vi "Find Edge Parameter.vi"(7 "Action":T6, 8 "error in (no error)":errorcluster, 9 "Line Fit Options in":T4={"Number of Lines"=1, "Type"=enum."First Edge Rake", "Min. Score"=10.0, "Max. Score"=1000.0, "Orientation"=0.0, "Angle Range"=45.0, "Angle Tolerance"=1.0, "Step Size"=7, "Min. SNR (db)"=0.0, "Min. Points (%)"=25.0, "Hough Iterations"=5} {"Min. Points (%)" min=0.0 max=100.0; "Min. SNR (db)" min=0.0; "Max. Score" min=0.0 max=1024.0; "Min. Score" min=0.0 max=1024.0 step=1.0}, 10 "Options in":T3={"Search Direction"=0, "Edge Options"={"Edge Polarity"=0, "Kernel Size"=3, "Width"=3, "Minimum Edge Strength"=10.0, "Interpolation Type"=enum."Bilinear Fixed", "Data Processing Method"=enum."Average"}, "Show Search Area"=FALSE, "Show Search Lines"=FALSE, "Show Edges Found"=FALSE, "Show Result"=TRUE, "Search Area Color"=65280, "Search Lines Color"=255, "Edge Locations Color"=16776960, "Result Color"=16711680, "Overlay Group Name"=""} {"Edge Options"."Edge Polarity" items=["All Edges", "Rising Edges", "Falling Edges"]; "Edge Options"."Minimum Edge Strength" format="%.2f"; "Edge Options"."Width" step=2; "Edge Options"."Kernel Size" step=2; "Search Direction" items=["Left to Right", "Right to Left", "Top to Bottom", "Bottom to Top"]}, 11 "Directory":string) -> (0 "error out":errorcluster, 2 "Line Fit Options out":T4={"Number of Lines"=1, "Type"=enum."First Edge Rake", "Min. Score"=10.0, "Max. Score"=1000.0, "Orientation"=0.0, "Angle Range"=45.0, "Angle Tolerance"=1.0, "Step Size"=7, "Min. SNR (db)"=0.0, "Min. Points (%)"=25.0, "Hough Iterations"=5} {"Min. Points (%)" min=0.0 max=100.0; "Min. SNR (db)" min=0.0; "Max. Score" min=0.0 max=1024.0; "Min. Score" min=0.0 max=1024.0 step=1.0}, 3 "Options out":T3={"Search Direction"=0, "Edge Options"={"Edge Polarity"=0, "Kernel Size"=3, "Width"=3, "Minimum Edge Strength"=10.0, "Interpolation Type"=enum."Bilinear Fixed", "Data Processing Method"=enum."Average"}, "Show Search Area"=FALSE, "Show Search Lines"=FALSE, "Show Edges Found"=FALSE, "Show Result"=TRUE, "Search Area Color"=65280, "Search Lines Color"=255, "Edge Locations Color"=16776960, "Result Color"=16711680, "Overlay Group Name"=""} {"Edge Options"."Edge Polarity" items=["All Edges", "Rising Edges", "Falling Edges"]; "Edge Options"."Minimum Edge Strength" format="%.2f"; "Edge Options"."Width" step=2; "Edge Options"."Kernel Size" step=2; "Search Direction" items=["Left to Right", "Right to Left", "Top to Bottom", "Bottom to Top"]})   [LabVIEW 2017, in "File.lvlib"]
uses:
  File.lvlib
  <vilib>/vision/Measure.llb/Edge Polarity.ctl
  <vilib>/vision/Measure.llb/Edge Options.ctl
  <vilib>/vision/Measure.llb/Straight Edge Process.ctl
  <vilib>/vision/Measure.llb/Straight Edge Options.ctl
  <vilib>/Utility/config.llb/NI_LVConfig.lvlib
  <vilib>/Utility/config.llb/Config Data RefNum.ctl
  <vilib>/Utility/config.llb/Read Key (Boolean).vi
  <vilib>/Utility/config.llb/Read Key (Double).vi
  <vilib>/Utility/config.llb/Read Key (U32).vi
  <vilib>/Utility/config.llb/Read Key (String).vi
  <vilib>/Utility/config.llb/Write Key (Boolean).vi
  <vilib>/Utility/config.llb/Write Key (Double).vi
  <vilib>/Utility/config.llb/Write Key (U32).vi
  <vilib>/Utility/config.llb/Write Key (String).vi
  Control/File Action.ctl
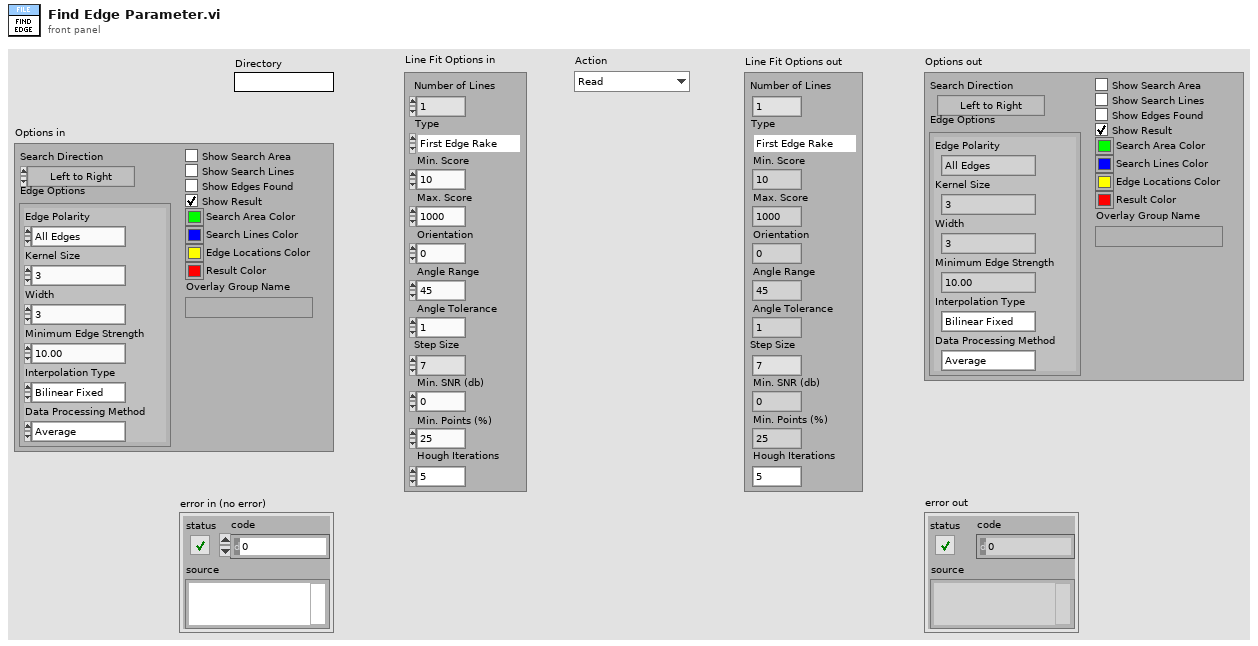
[diagram p1: front panel]
types:
  T1 = typedef "Edge Options.ctl" = cluster{"Edge Polarity":T2, "Kernel Size":u32, "Width":u32, "Minimum Edge Strength":sgl, "Interpolation Type":enum32{"Zero Order", "Bilinear", "Quadratic", "Cubic", "Bilinear Fixed"}, "Data Processing Method":enum32{"Average", "Median"}}
  T2 = typedef "Edge Polarity.ctl" = u32
  T3 = cluster{"Search Direction":u32, "Edge Options":T1, "Show Search Area":bool, "Show Search Lines":bool, "Show Edges Found":bool, "Show Result":bool, "Search Area Color":u32, "Search Lines Color":u32, "Edge Locations Color":u32, "Result Color":u32, "Overlay Group Name":string}
  T4 = typedef "Straight Edge Options.ctl" = cluster{"Number of Lines":i32, "Type":T5, "Min. Score":dbl, "Max. Score":dbl, "Orientation":dbl, "Angle Range":dbl, "Angle Tolerance":dbl, "Step Size":u32, "Min. SNR (db)":dbl, "Min. Points (%)":dbl, "Hough Iterations":i32}
  T5 = typedef "Straight Edge Process.ctl" = enum32{"First Edge Rake", "Best Edge Rake", "Hough Edge Rake", "First Edge Projection", "Best Edge Projection"}
  T6 = typedef "File.lvlib/File Action.ctl" = enum16{"Read", "Write"}
  T7 = typedef "NI_LVConfig.lvlib/Config Data RefNum.ctl" = refnum<k1>
  T8 = cluster{"Config refnum":T7, "Options":cluster{"Search Direction":u32, "Edge Options":T1, "Show Search Area":bool, "Show Search Lines":bool, "Show Edges Found":bool, "Show Result":bool, "Search Area Color":u32, "Search Lines Color":u32, "Edge Locations Color":u32, "Result Color":u32, "Overlay Group Name":string}, "Line Fit Options":T4, "Section":cluster{"Options":string, "Line Fit Options":string}}
  T9 = enum32{"Zero Order", "Bilinear", "Quadratic", "Cubic", "Bilinear Fixed"}
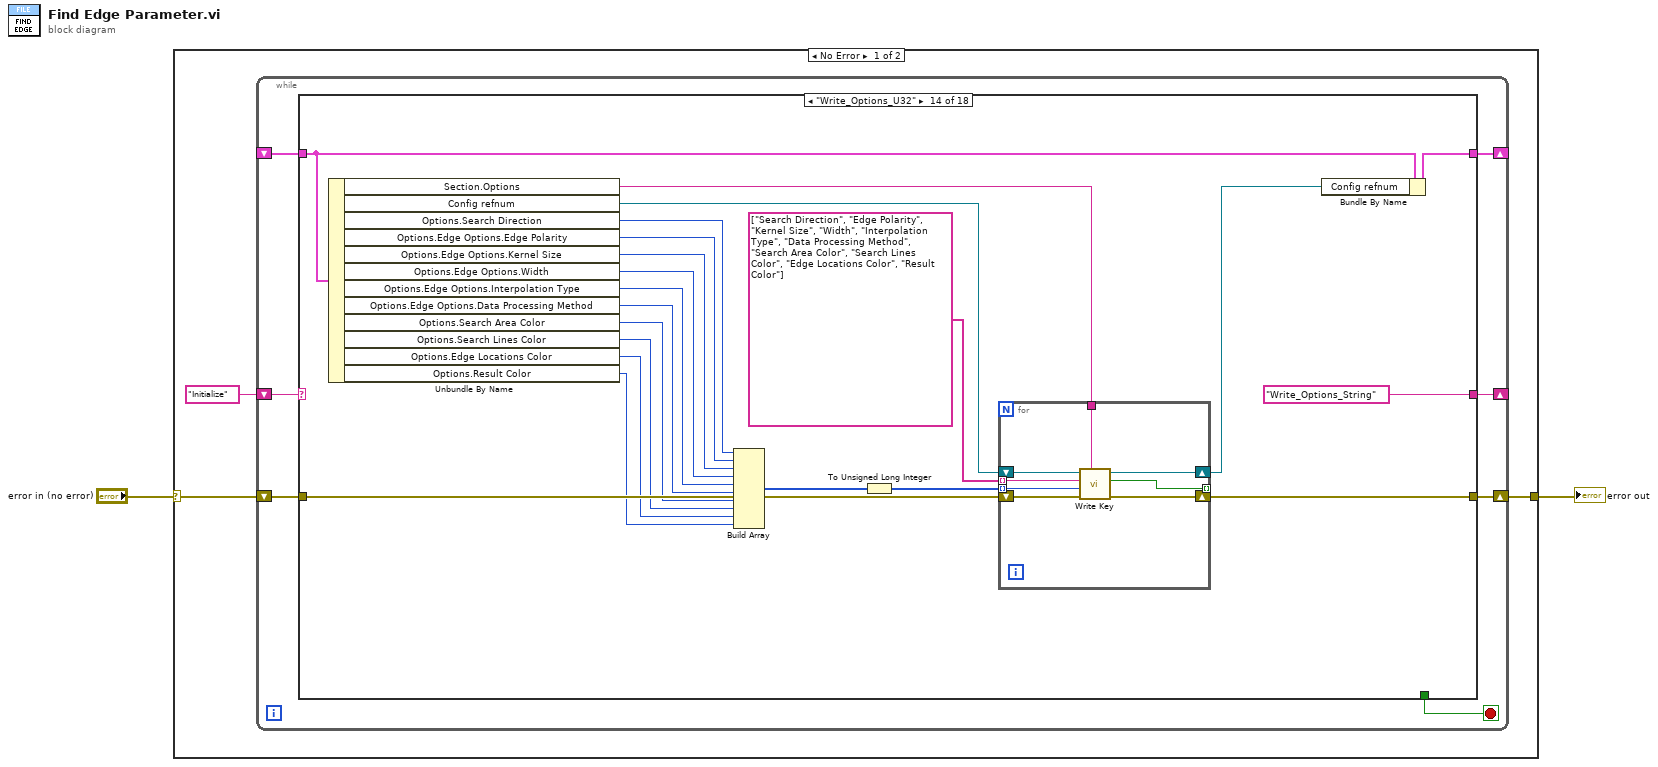
[diagram p0: block diagram]
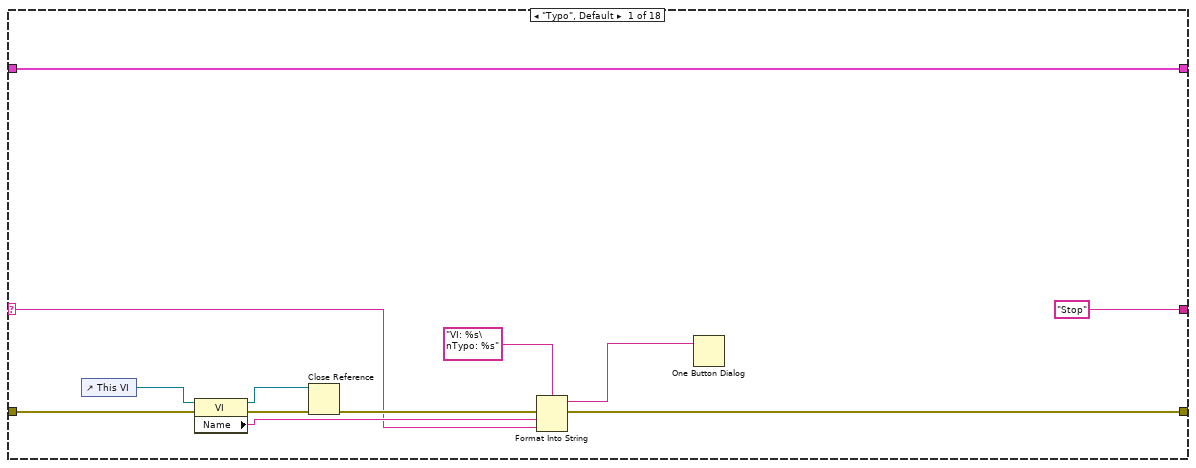
[diagram p2: hidden frame]
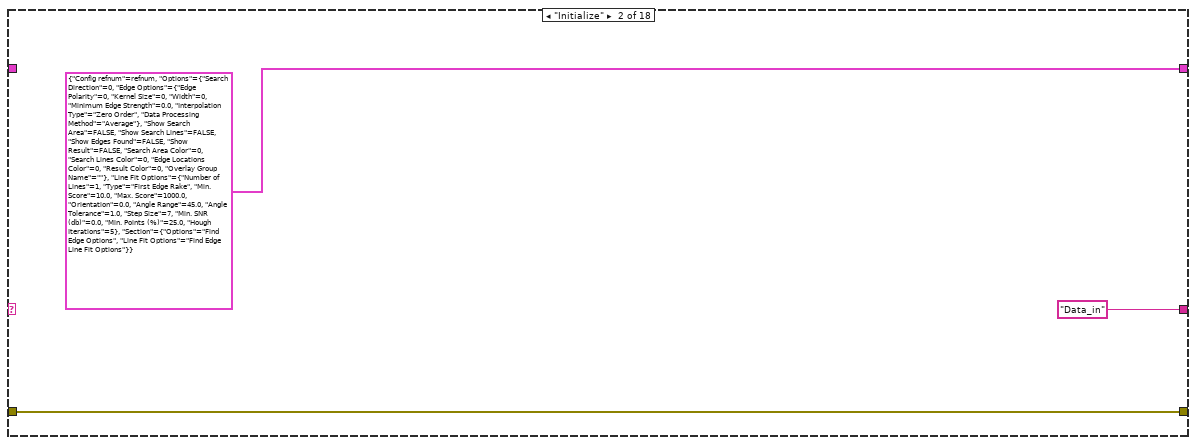
[diagram p3: hidden frame]
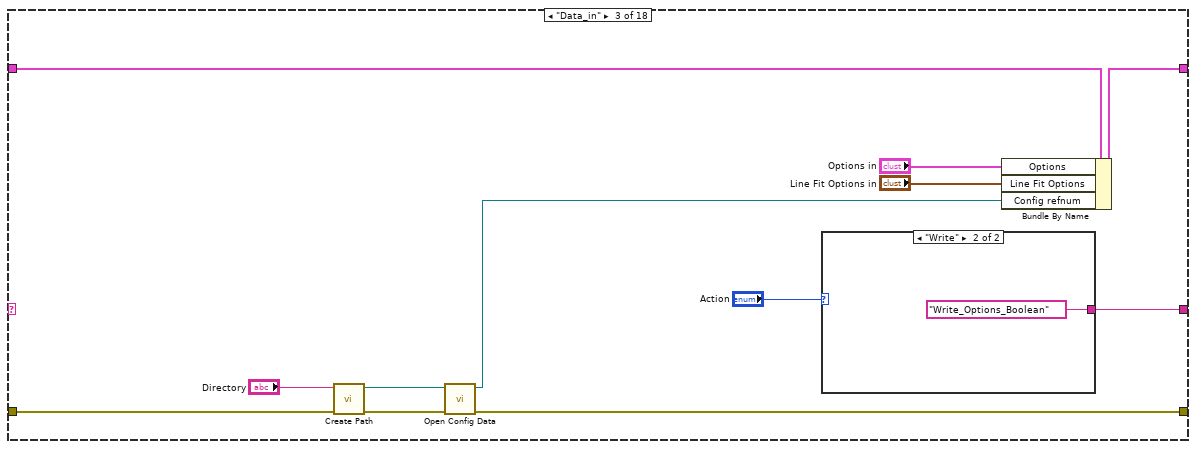
[diagram p4: hidden frame]
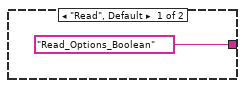
[diagram p5: hidden frame]
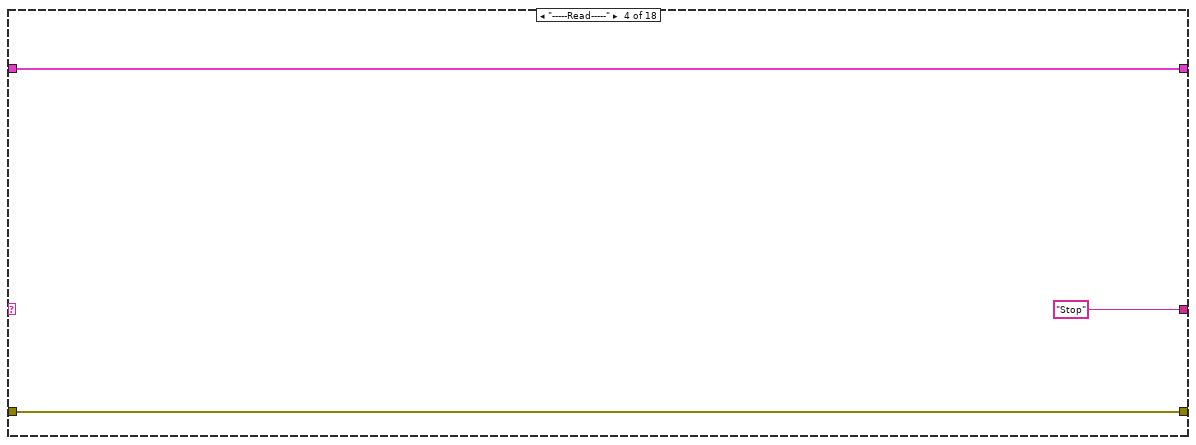
[diagram p6: hidden frame]
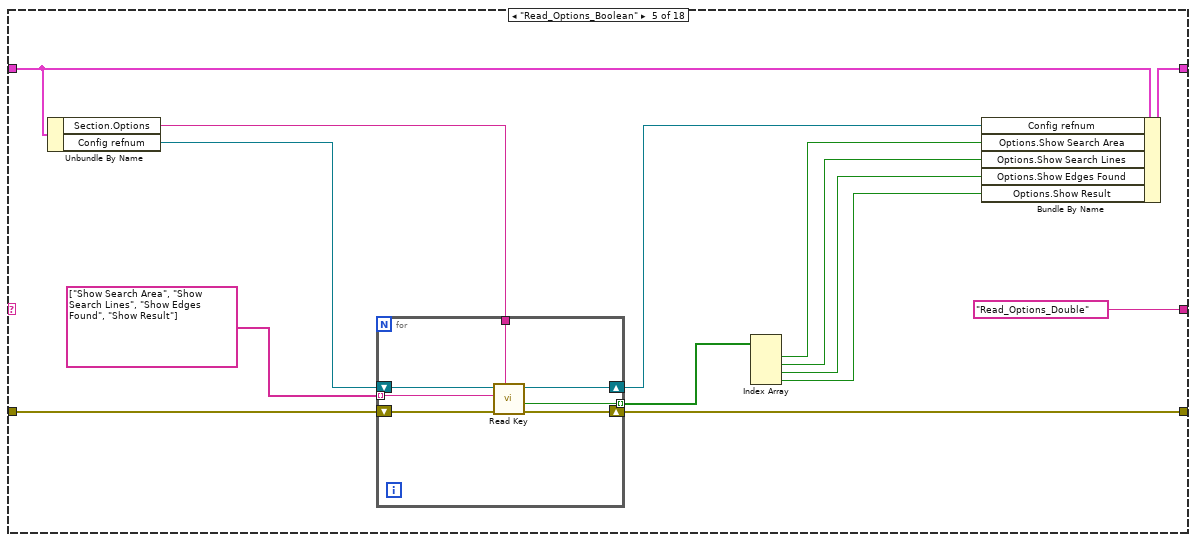
[diagram p7: hidden frame]
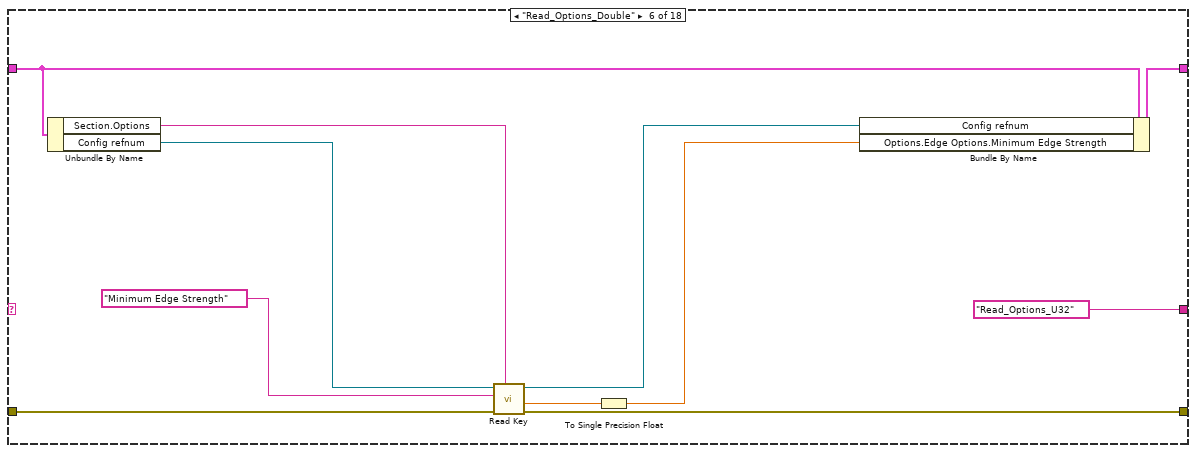
[diagram p8: hidden frame]
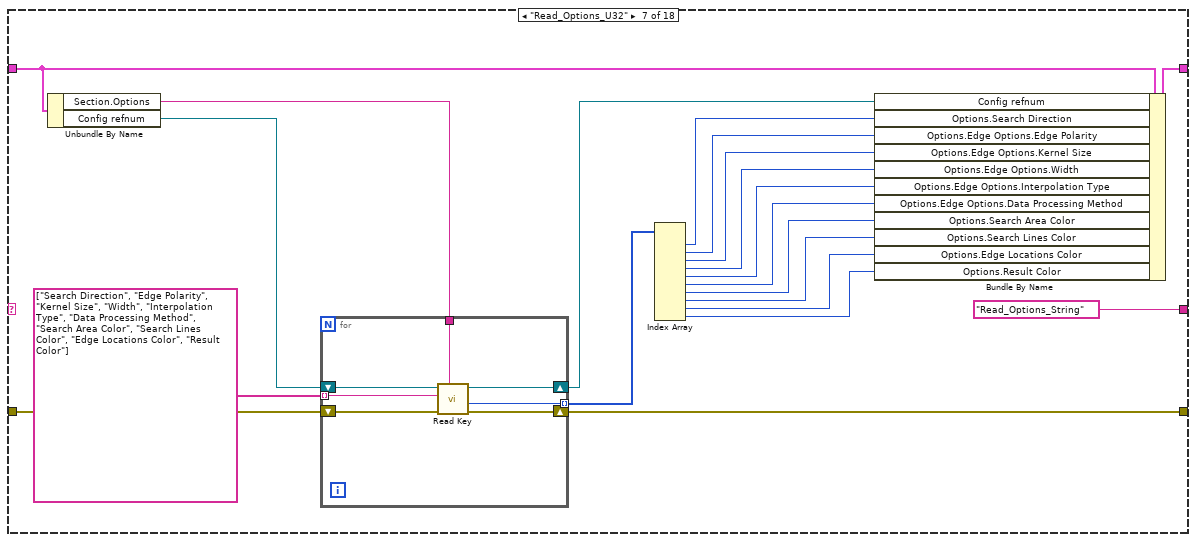
[diagram p9: hidden frame]
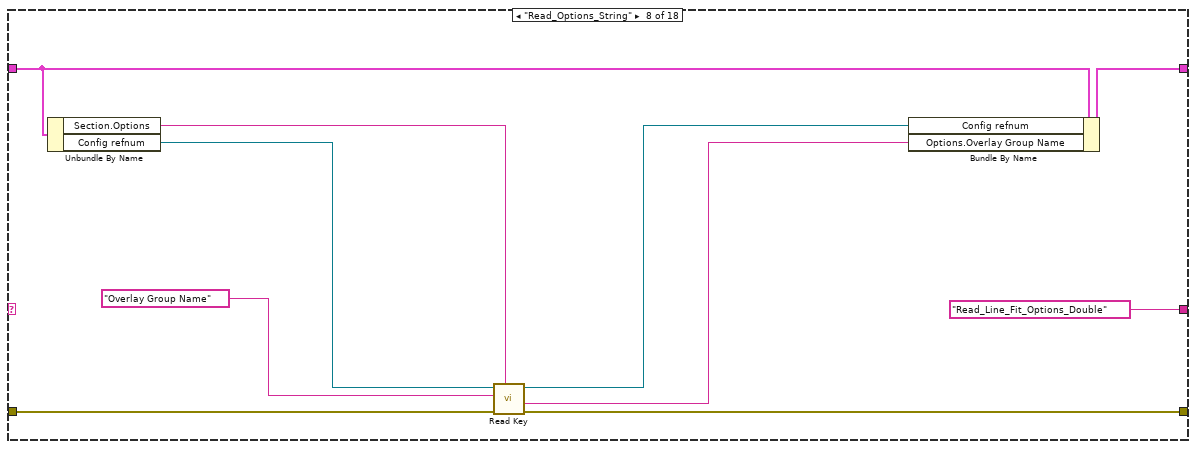
[diagram p10: hidden frame]
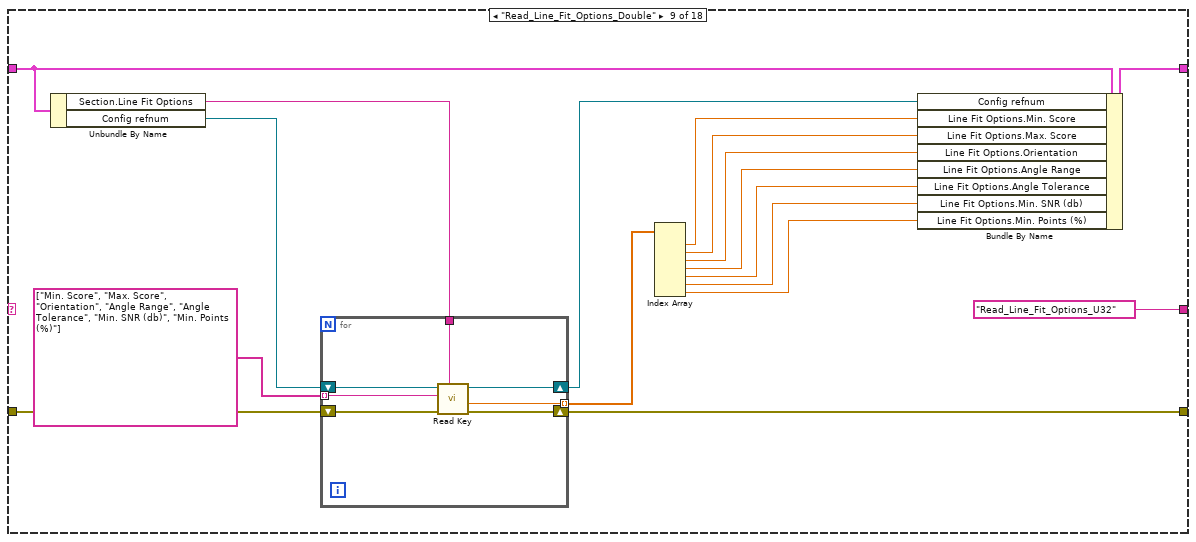
[diagram p11: hidden frame]
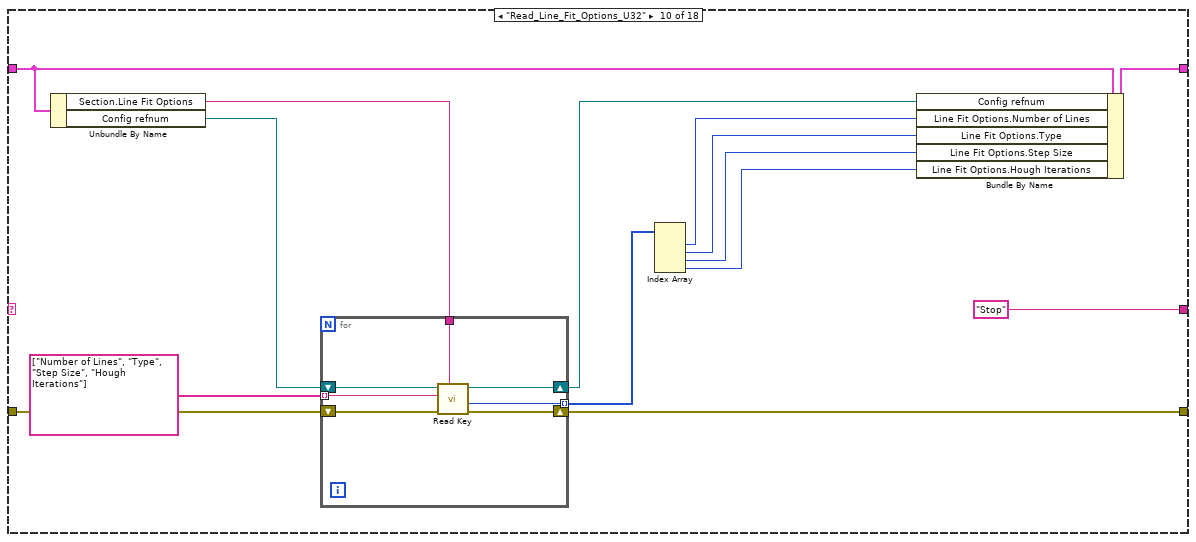
[diagram p12: hidden frame]
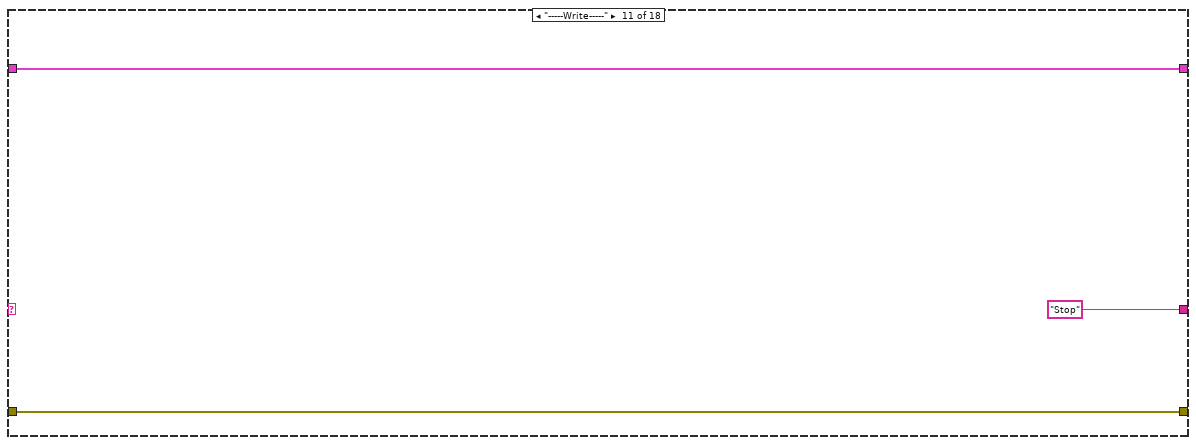
[diagram p13: hidden frame]
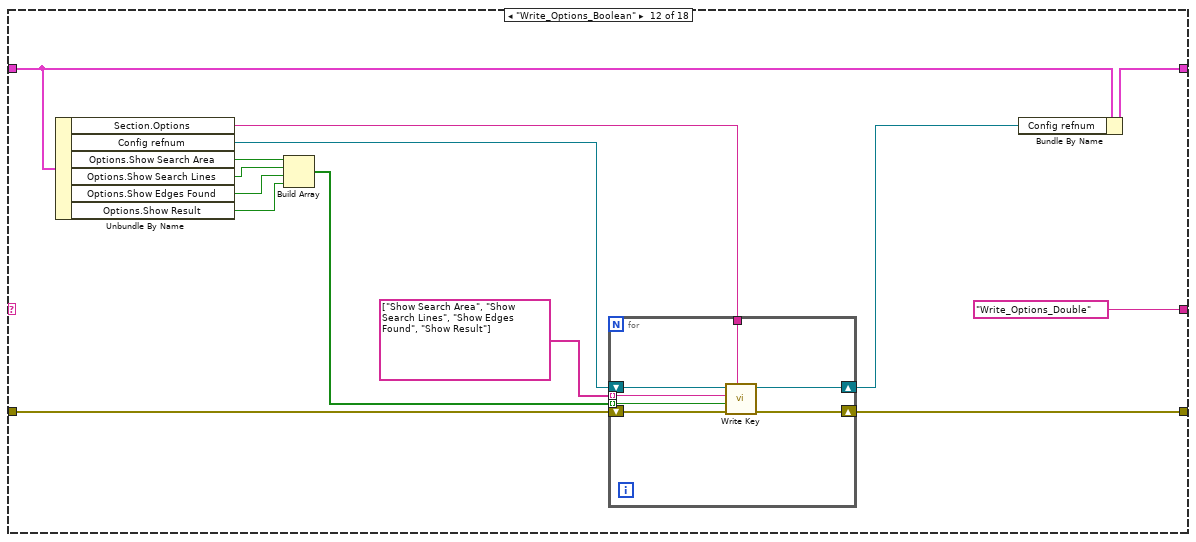
[diagram p14: hidden frame]
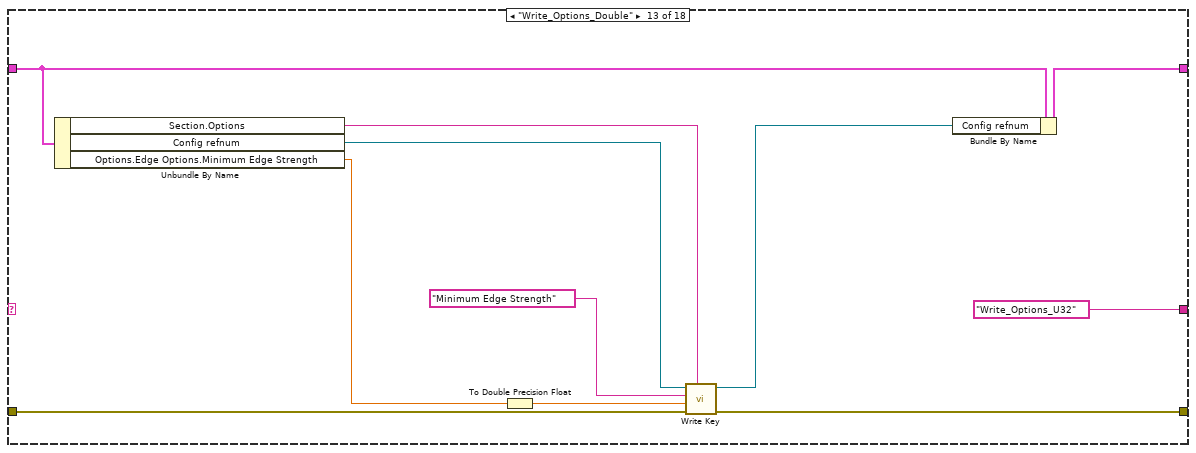
[diagram p15: hidden frame]
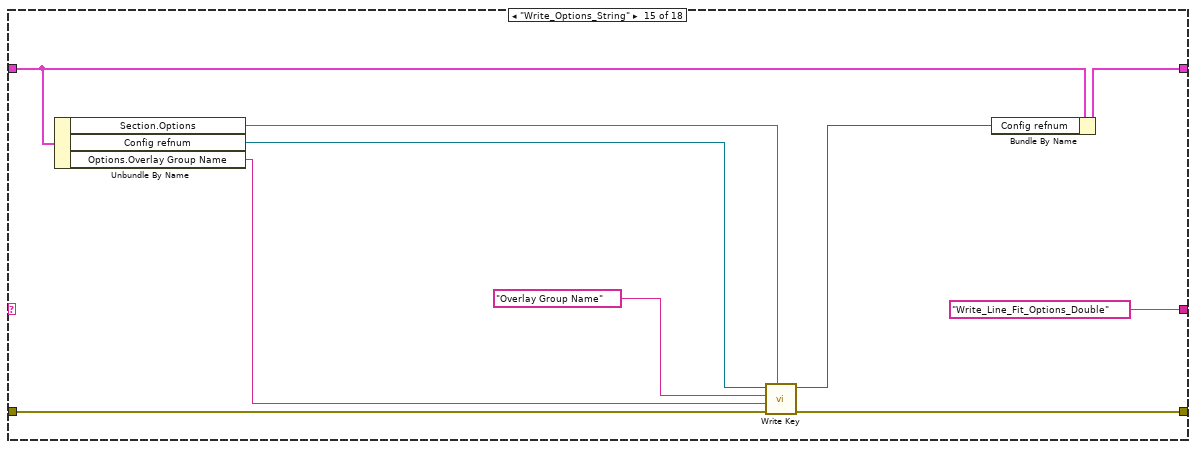
[diagram p16: hidden frame]
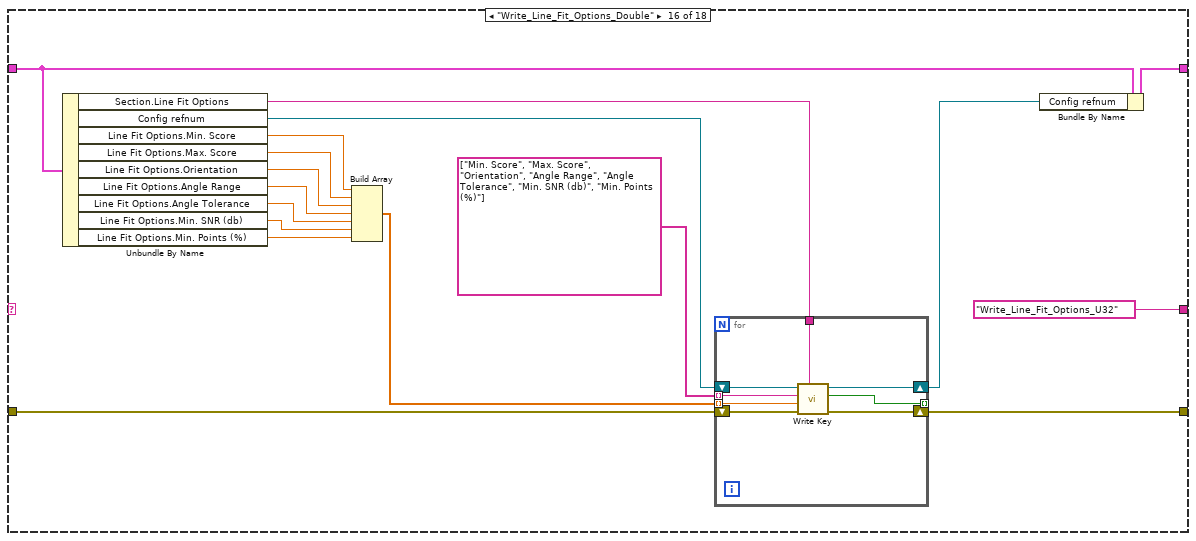
[diagram p17: hidden frame]
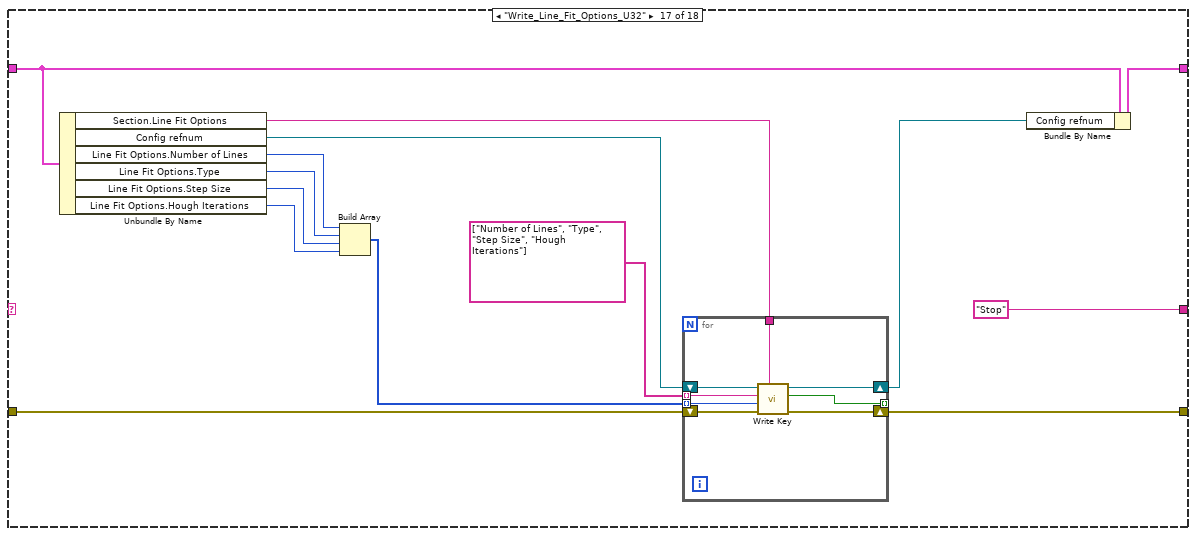
[diagram p18: hidden frame]
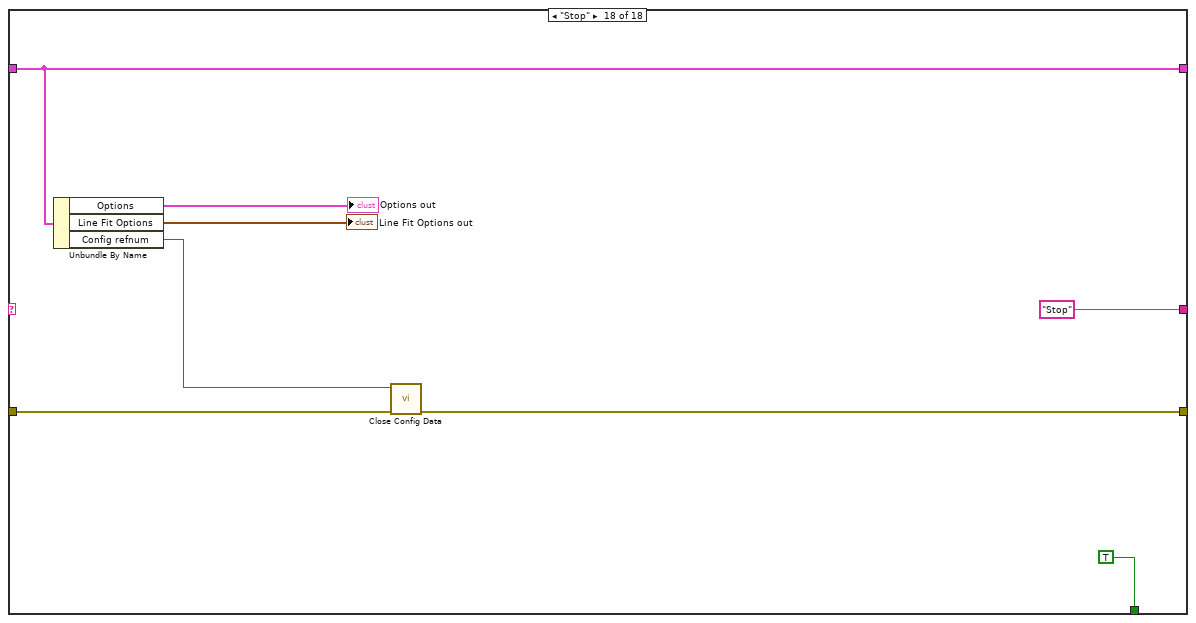
[diagram p19: hidden frame]
diagram:
  n1 = case shown="No Error" "error in (no error)" {
    selector: "error in (no error)" -> [w5 w288]
    tunnel: [w3 w288] -> w1
    frame No Error {
      n2 = while {
        shift-right: [w10] -> w3
        shift-left: w5 -> [w11]
        shift-right: [w9] -> _
        shift-left: "Initialize" -> [w12]
        shift-right: [w7] -> _
        shift-left: _ -> [w6]
        stop <- w8 stop-if-true
        n3 = case shown="\"Write_Options_U32\"" w12 {
          selector: w12 -> [w16 _ _ _ _ _ _ _ _ _ _ _ _ _ _ _ _ _]
          tunnel: w11 -> [w24 w26 w39 w44 w58 w76 w96 w113 w130 w151 w161 w175 w193 w214 w232 w249 w271 w285]
          tunnel: [w21 w26 w34 w44 w56 w74 w94 w111 w128 w149 w161 w173 w191 w212 w230 w247 w269 w283] -> w10
          tunnel: ["Stop" "Data_in" w36 "Stop" "Read_Options_Double" "Read_Options_U32" "Read_Options_String" "Read_Line_Fit_Options_Double" "Read_Line_Fit_Options_U32" "Stop" "Stop" "Write_Options_Double" "Write_Options_U32" "Write_Options_String" "Write_Line_Fit_Options_Double" "Write_Line_Fit_Options_U32" "Stop" "Stop"] -> w9
          tunnel: [_ _ _ _ _ _ _ _ _ _ _ _ _ _ _ _ _ TRUE] -> w8
          tunnel: [w13 T8 {"Config refnum"=refnum, "Options"={"Search Direction"=0, "Edge Options"={"Edge Polarity"=0, "Kernel Size"=0, "Width"=0, "Minimum Edge Strength"=0.0, "Interpolation Type"=enum."Zero Order", "Data Processing Method"=enum."Average"}, "Show Search Area"=FALSE, "Show Search Lines"=FALSE, "Show Edges Found"=FALSE, "Show Result"=FALSE, "Search Area Color"=0, "Search Lines Color"=0, "Edge Locations Color"=0, "Result Color"=0, "Overlay Group Name"=""}, "Line Fit Options"={"Number of Lines"=1, "Type"=enum."First Edge Rake", "Min. Score"=10.0, "Max. Score"=1000.0, "Orientation"=0.0, "Angle Range"=45.0, "Angle Tolerance"=1.0, "Step Size"=7, "Min. SNR (db)"=0.0, "Min. Points (%)"=25.0, "Hough Iterations"=5}, "Section"={"Options"="Find Edge Options", "Line Fit Options"="Find Edge Line Fit Options"}} w37 w43 w51 w70 w89 w107 w123 w144 w160 w169 w187 w208 w226 w243 w265 w284] -> w7
          tunnel: w6 -> [w13 _ w38 w43 w57 w75 w95 w112 w129 w150 w160 w174 w192 w213 w231 w248 w270 w284]
          frame "Typo", Default {
            n4 = control-ref of="This VI"() -> (w22:refnum<vi>)
            n5 = property class="VI"(reference=w22, error in=w24) -> (reference out=w17:refnum<vi>, error out=w23:errorcluster, "Name"=w19:string)
            n6 = Close Reference(reference=w17, error in (no error)=w23) -> (error out=w18:errorcluster)
            n7 = Format Into String(format string="VI: %s\nTypo: %s", error in=w18, w19, w16) -> (resulting string=w15:string, error out=w21:errorcluster)  [unwired: 1 in]
            n8 = One Button Dialog(message=w15) -> ()  [unwired: 1 in, 1 out]
          }
          frame "Initialize" {
          }
          frame "Data_in" {
            n9 = call "Create Path.vi"("error in (no error)"=w39, "Directory"="Directory") -> ("error out"=w35:errorcluster, "Path"=w33:path)  [unwired: 8 in]
            n10 = call <vilib>:"Open Config Data.vi"("error in (no error)"=w35, "configuration file path"=w33) -> ("error out"=w34:errorcluster, "refnum"=w31:T7)  [unwired: 7 in, 1 out]
            n11 = case shown="\"Write\"" "Action" {
              tunnel: ["Read_Options_Boolean" "Write_Options_Boolean"] -> w36
              frame "Read", Default {
              }
              frame "Write" {
              }
            }
            n12 = Bundle By Name(cluster=w38, "Options"="Options in", "Line Fit Options"="Line Fit Options in", "Config refnum"=w31) -> (w37:T8)
          }
          frame "-----Read-----" {
          }
          frame "Read_Options_Boolean" {
            n13 = Unbundle By Name(w57) -> ("Section.Options"=w55:string, "Config refnum"=w54:T7)
            n14 = for {
              tunnel: w55 -> [w63]
              shift-right: [w64] -> w56
              shift-left: w58 -> [w65]
              shift-right: [w61] -> w50
              shift-left: w54 -> [w62]
              tunnel: string[] ["Show Search Area", "Show Search Lines", "Show Edges Found", "Show Result"] -> [w60] mode=indexing
              tunnel: [w59] -> w52 mode=indexing
              n15 = call-poly <vilib>:"Read Key.vi"("section"=w63, "error in (no error)"=w65, "key"=w60, "refnum"=w62) -> ("error out"=w64:errorcluster, "value"=w59:bool, "refnum out"=w61:T7)  [unwired: 4 in, 1 out]
            }
            n16 = Index Array(array=w52) -> (element #1=w49:bool, element #2=w48:bool, element #3=w47:bool, element #4=w46:bool)  [unwired: 4 in]
            n17 = Bundle By Name(cluster=w57, "Config refnum"=w50, "Options.Show Search Area"=w49, "Options.Show Search Lines"=w48, "Options.Show Edges Found"=w47, "Options.Show Result"=w46) -> (w51:T8)
          }
          frame "Read_Options_Double" {
            n18 = Unbundle By Name(w75) -> ("Section.Options"=w73:string, "Config refnum"=w72:T7)
            n19 = call-poly <vilib>:"Read Key.vi"("section"=w73, "error in (no error)"=w76, "key"="Minimum Edge Strength", "refnum"=w72) -> ("error out"=w74:errorcluster, "value"=w67:dbl, "refnum out"=w69:T7)  [unwired: 4 in, 1 out]
            n20 = To Single Precision Float(number=w67) -> (single precision float=w66:sgl)
            n21 = Bundle By Name(cluster=w75, "Config refnum"=w69, "Options.Edge Options.Minimum Edge Strength"=w66) -> (w70:T8)
          }
          frame "Read_Options_U32" {
            n22 = Unbundle By Name(w95) -> ("Section.Options"=w93:string, "Config refnum"=w92:T7)
            n23 = for {
              tunnel: w93 -> [w101]
              shift-right: [w102] -> w94
              shift-left: w96 -> [w103]
              shift-right: [w99] -> w88
              shift-left: w92 -> [w100]
              tunnel: string[] ["Search Direction", "Edge Polarity", "Kernel Size", "Width", "Interpolation Type", "Data Processing Method", "Search Area Color", "Search Lines Color", "Edge Locations Color", "Result Color"] -> [w98] mode=indexing
              tunnel: [w97] -> w90 mode=indexing
              n24 = call-poly <vilib>:"Read Key.vi"("section"=w101, "error in (no error)"=w103, "key"=w98, "refnum"=w100) -> ("error out"=w102:errorcluster, "value"=w97:u32, "refnum out"=w99:T7)  [unwired: 4 in, 1 out]
            }
            n25 = Index Array(array=w90) -> (element #1=w87:u32, element #2=w86:u32, element #3=w85:u32, element #4=w84:u32, element #5=w82:u32, element #6=w81:u32, element #7=w80:u32, element #8=w79:u32, element #9=w78:u32, element #10=w77:u32)  [unwired: 10 in]
            n26 = Bundle By Name(cluster=w95, "Config refnum"=w88, "Options.Search Direction"=w87, "Options.Edge Options.Edge Polarity"=w86, "Options.Edge Options.Kernel Size"=w85, "Options.Edge Options.Width"=w84, "Options.Edge Options.Interpolation Type"=w82, "Options.Edge Options.Data Processing Method"=w81, "Options.Search Area Color"=w80, "Options.Search Lines Color"=w79, "Options.Edge Locations Color"=w78, "Options.Result Color"=w77) -> (w89:T8)
          }
          frame "Read_Options_String" {
            n27 = Unbundle By Name(w112) -> ("Section.Options"=w110:string, "Config refnum"=w109:T7)
            n28 = call-poly <vilib>:"Read Key.vi"("section"=w110, "error in (no error)"=w113, "key"="Overlay Group Name", "refnum"=w109) -> ("error out"=w111:errorcluster, "value"=w104:string, "refnum out"=w106:T7)  [unwired: 4 in, 1 out]
            n29 = Bundle By Name(cluster=w112, "Config refnum"=w106, "Options.Overlay Group Name"=w104) -> (w107:T8)
          }
          frame "Read_Line_Fit_Options_Double" {
            n30 = Unbundle By Name(w129) -> ("Section.Line Fit Options"=w127:string, "Config refnum"=w126:T7)
            n31 = for {
              tunnel: w127 -> [w135]
              shift-right: [w136] -> w128
              shift-left: w130 -> [w137]
              shift-right: [w133] -> w122
              shift-left: w126 -> [w134]
              tunnel: string[] ["Min. Score", "Max. Score", "Orientation", "Angle Range", "Angle Tolerance", "Min. SNR (db)", "Min. Points (%)"] -> [w132] mode=indexing
              tunnel: [w131] -> w124 mode=indexing
              n32 = call-poly <vilib>:"Read Key.vi"("section"=w135, "error in (no error)"=w137, "key"=w132, "refnum"=w134) -> ("error out"=w136:errorcluster, "value"=w131:dbl, "refnum out"=w133:T7)  [unwired: 4 in, 1 out]
            }
            n33 = Index Array(array=w124) -> (element #1=w121:dbl, element #2=w120:dbl, element #3=w119:dbl, element #4=w118:dbl, element #5=w116:dbl, element #6=w115:dbl, element #7=w114:dbl)  [unwired: 7 in]
            n34 = Bundle By Name(cluster=w129, "Config refnum"=w122, "Line Fit Options.Min. Score"=w121, "Line Fit Options.Max. Score"=w120, "Line Fit Options.Orientation"=w119, "Line Fit Options.Angle Range"=w118, "Line Fit Options.Angle Tolerance"=w116, "Line Fit Options.Min. SNR (db)"=w115, "Line Fit Options.Min. Points (%)"=w114) -> (w123:T8)
          }
          frame "Read_Line_Fit_Options_U32" {
            n35 = Unbundle By Name(w150) -> ("Section.Line Fit Options"=w148:string, "Config refnum"=w147:T7)
            n36 = for {
              tunnel: w148 -> [w156]
              shift-right: [w157] -> w149
              shift-left: w151 -> [w158]
              shift-right: [w154] -> w143
              shift-left: w147 -> [w155]
              tunnel: string[] ["Number of Lines", "Type", "Step Size", "Hough Iterations"] -> [w153] mode=indexing
              tunnel: [w152] -> w145 mode=indexing
              n37 = call-poly <vilib>:"Read Key.vi"("section"=w156, "error in (no error)"=w158, "key"=w153, "refnum"=w155) -> ("error out"=w157:errorcluster, "value"=w152:u32, "refnum out"=w154:T7)  [unwired: 4 in, 1 out]
            }
            n38 = Index Array(array=w145) -> (element #1=w142:u32, element #2=w141:u32, element #3=w140:u32, element #4=w139:u32)  [unwired: 4 in]
            n39 = Bundle By Name(cluster=w150, "Config refnum"=w143, "Line Fit Options.Number of Lines"=w142, "Line Fit Options.Type"=w141, "Line Fit Options.Step Size"=w140, "Line Fit Options.Hough Iterations"=w139) -> (w144:T8)
          }
          frame "-----Write-----" {
          }
          frame "Write_Options_Boolean" {
            n40 = Unbundle By Name(w174) -> ("Section.Options"=w172:string, "Config refnum"=w171:T7, "Options.Show Search Area"=w166:bool, "Options.Show Search Lines"=w165:bool, "Options.Show Edges Found"=w163:bool, "Options.Show Result"=w164:bool)
            n41 = Build Array(w166, w165, w163, w164) -> (w162:bool[])
            n42 = for {
              tunnel: w172 -> [w180]
              shift-right: [w181] -> w173
              shift-left: w175 -> [w182]
              shift-right: [w178] -> w168
              shift-left: w171 -> [w179]
              tunnel: string[] ["Show Search Area", "Show Search Lines", "Show Edges Found", "Show Result"] -> [w177] mode=indexing
              tunnel: w162 -> [w176] mode=indexing
              n43 = call-poly <vilib>:"Write Key.vi"("section"=w180, "error in (no error)"=w182, "value"=w176, "key"=w177, "refnum"=w179) -> ("error out"=w181:errorcluster, "refnum out"=w178:T7)  [unwired: 4 in, 1 out]
            }
            n44 = Bundle By Name(cluster=w174, "Config refnum"=w168) -> (w169:T8)
          }
          frame "Write_Options_Double" {
            n45 = Unbundle By Name(w192) -> ("Section.Options"=w190:string, "Config refnum"=w189:T7, "Options.Edge Options.Minimum Edge Strength"=w184:sgl)
            n46 = To Double Precision Float(number=w184) -> (double precision float=w183:dbl)
            n47 = call-poly <vilib>:"Write Key.vi"("section"=w190, "error in (no error)"=w193, "value"=w183, "key"="Minimum Edge Strength", "refnum"=w189) -> ("error out"=w191:errorcluster, "refnum out"=w186:T7)  [unwired: 4 in, 1 out]
            n48 = Bundle By Name(cluster=w192, "Config refnum"=w186) -> (w187:T8)
          }
          frame "Write_Options_U32" {
            n49 = Unbundle By Name(w213) -> ("Section.Options"=w211:string, "Config refnum"=w210:T7, "Options.Search Direction"=w205:u32, "Options.Edge Options.Edge Polarity"=w204:T2, "Options.Edge Options.Kernel Size"=w203:u32, "Options.Edge Options.Width"=w202:u32, "Options.Edge Options.Interpolation Type"=w201:T9, "Options.Edge Options.Data Processing Method"=w200:enum32{"Average", "Median"}, "Options.Search Area Color"=w199:u32, "Options.Search Lines Color"=w198:u32, "Options.Edge Locations Color"=w197:u32, "Options.Result Color"=w196:u32)
            n50 = Build Array(w205, w204, w203, w202, w201, w200, w199, w198, w197, w196) -> (w195:T2[])
            n51 = To Unsigned Long Integer(number=w195) -> (unsigned 32bit integer=w194:T2[])
            n52 = for {
              tunnel: w211 -> [w220]
              shift-right: [w221] -> w212
              shift-left: w214 -> [w222]
              shift-right: [w218] -> w207
              shift-left: w210 -> [w219]
              tunnel: string[] ["Search Direction", "Edge Polarity", "Kernel Size", "Width", "Interpolation Type", "Data Processing Method", "Search Area Color", "Search Lines Color", "Edge Locations Color", "Result Color"] -> [w217] mode=indexing
              tunnel: [w216] -> _ mode=indexing
              tunnel: w194 -> [w215] mode=indexing
              n53 = call-poly <vilib>:"Write Key.vi"("section"=w220, "error in (no error)"=w222, "value"=w215, "key"=w217, "refnum"=w219) -> ("error out"=w221:errorcluster, "found?"=w216:bool, "refnum out"=w218:T7)  [unwired: 4 in]
            }
            n54 = Bundle By Name(cluster=w213, "Config refnum"=w207) -> (w208:T8)
          }
          frame "Write_Options_String" {
            n55 = Unbundle By Name(w231) -> ("Section.Options"=w229:string, "Config refnum"=w228:T7, "Options.Overlay Group Name"=w223:string)
            n56 = call-poly <vilib>:"Write Key.vi"("section"=w229, "error in (no error)"=w232, "value"=w223, "key"="Overlay Group Name", "refnum"=w228) -> ("error out"=w230:errorcluster, "refnum out"=w225:T7)  [unwired: 4 in, 1 out]
            n57 = Bundle By Name(cluster=w231, "Config refnum"=w225) -> (w226:T8)
          }
          frame "Write_Line_Fit_Options_Double" {
            n58 = Unbundle By Name(w248) -> ("Section.Line Fit Options"=w246:string, "Config refnum"=w245:T7, "Line Fit Options.Min. Score"=w240:dbl, "Line Fit Options.Max. Score"=w239:dbl, "Line Fit Options.Orientation"=w238:dbl, "Line Fit Options.Angle Range"=w237:dbl, "Line Fit Options.Angle Tolerance"=w236:dbl, "Line Fit Options.Min. SNR (db)"=w235:dbl, "Line Fit Options.Min. Points (%)"=w234:dbl)
            n59 = Build Array(w240, w239, w238, w237, w236, w235, w234) -> (w233:dbl[])
            n60 = for {
              tunnel: w246 -> [w255]
              shift-right: [w256] -> w247
              shift-left: w249 -> [w257]
              shift-right: [w253] -> w242
              shift-left: w245 -> [w254]
              tunnel: string[] ["Min. Score", "Max. Score", "Orientation", "Angle Range", "Angle Tolerance", "Min. SNR (db)", "Min. Points (%)"] -> [w252] mode=indexing
              tunnel: [w251] -> _ mode=indexing
              tunnel: w233 -> [w250] mode=indexing
              n61 = call-poly <vilib>:"Write Key.vi"("section"=w255, "error in (no error)"=w257, "value"=w250, "key"=w252, "refnum"=w254) -> ("error out"=w256:errorcluster, "found?"=w251:bool, "refnum out"=w253:T7)  [unwired: 4 in]
            }
            n62 = Bundle By Name(cluster=w248, "Config refnum"=w242) -> (w243:T8)
          }
          frame "Write_Line_Fit_Options_U32" {
            n63 = Unbundle By Name(w270) -> ("Section.Line Fit Options"=w268:string, "Config refnum"=w267:T7, "Line Fit Options.Number of Lines"=w262:i32, "Line Fit Options.Type"=w259:T5, "Line Fit Options.Step Size"=w260:u32, "Line Fit Options.Hough Iterations"=w261:i32)
            n64 = Build Array(w262, w259, w260, w261) -> (w258:u32[])
            n65 = for {
              tunnel: w268 -> [w277]
              shift-right: [w278] -> w269
              shift-left: w271 -> [w279]
              shift-right: [w275] -> w264
              shift-left: w267 -> [w276]
              tunnel: string[] ["Number of Lines", "Type", "Step Size", "Hough Iterations"] -> [w274] mode=indexing
              tunnel: [w273] -> _ mode=indexing
              tunnel: w258 -> [w272] mode=indexing
              n66 = call-poly <vilib>:"Write Key.vi"("section"=w277, "error in (no error)"=w279, "value"=w272, "key"=w274, "refnum"=w276) -> ("error out"=w278:errorcluster, "found?"=w273:bool, "refnum out"=w275:T7)  [unwired: 4 in]
            }
            n67 = Bundle By Name(cluster=w270, "Config refnum"=w264) -> (w265:T8)
          }
          frame "Stop" {
            n68 = Unbundle By Name(w284) -> ("Options"=→"Options out":T3, "Line Fit Options"=→"Line Fit Options out":T4, "Config refnum"=w282:T7)
            n69 = call <vilib>:"Close Config Data.vi"("error in (no error)"=w285, "refnum"=w282) -> ("error out"=w283:errorcluster)  [unwired: 8 in, 1 out]
          }
        }
      }
    }
    frame Error {
    }
  }
  "error out" <- w1
